vi "ReadALLControlRefs.vi"(8 "error in (no error)":errorcluster, 11 "CtlLookup In":T1) -> (0 "error out":errorcluster, 1 "CtlRef Array":refnum<vi>[](array[refnum]), 2 "CtlName Array":string[](array[string]), 3 "CtlLookup Out":T1)   [LabVIEW 2018, in "CtlReferences.lvlib" / "CtlReferences.lvclass"]
doc: "Read all Refs from DVR"
uses:
  CtlReferences.lvclass
  TypeDefs/CtlLookup.ctl
  CtlReferences.lvclass/CtlReferences.ctl
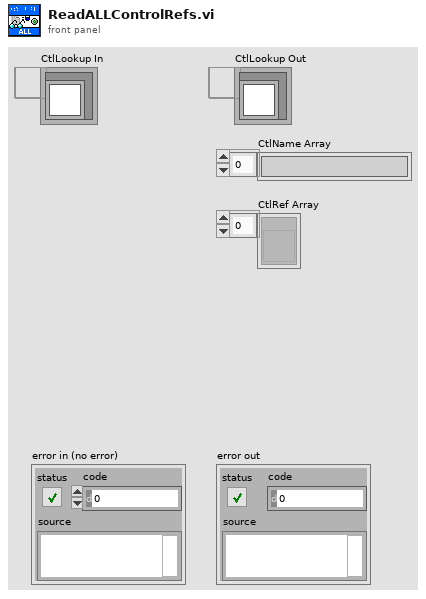
[diagram p1: front panel]
types:
  T1 = typedef "CtlReferences.lvlib/CtlReferences.lvclass/CtlLookup.ctl" = refnum<data-value>
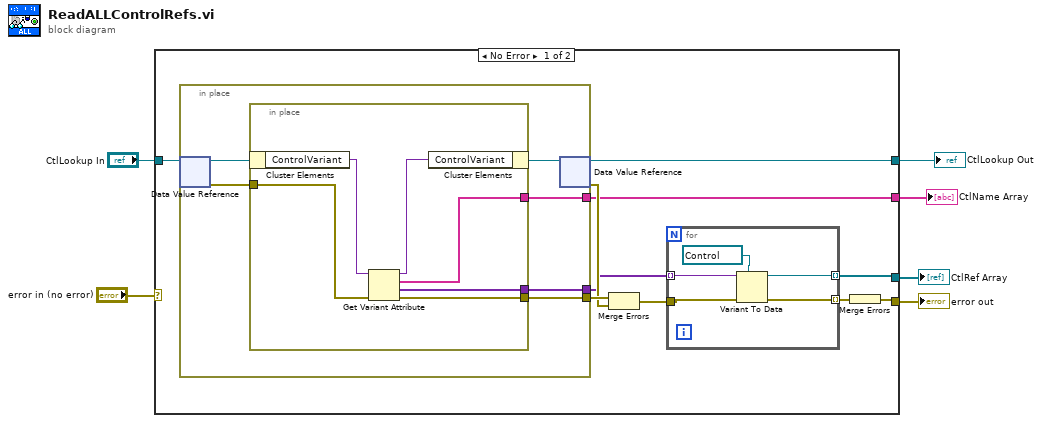
[diagram p0: block diagram]
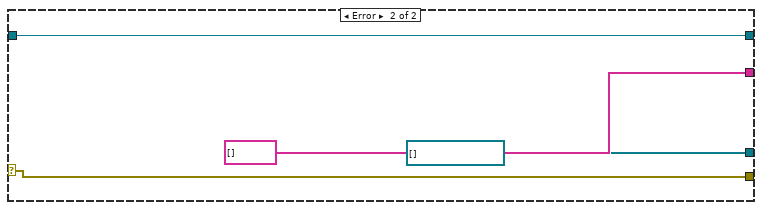
[diagram p2: hidden frame]
diagram:
  n1 = case shown="No Error" "error in (no error)" {
    selector: "error in (no error)" -> [_ w37]
    tunnel: "CtlLookup In" -> [w16 w35]
    tunnel: [w7 w37] -> w1
    tunnel: [w13 string[] []] -> w4
    tunnel: [w12 w35] -> w6
    tunnel: [w8 refnum<vi>[] []] -> w2
    frame No Error {
      n2 = in-place {
        in-place-border: [w26] -> w13
        in-place-border: [w25] -> w9
        in-place-border: [w24] -> w15
        n3 = in-place-dvr #1(w16) -> (w23:refnum<class "CtlReferences.lvclass">, w27:errorcluster)
        n4 = in-place {
          in-place-border: w27 -> [w33]
          in-place-border: [w32] -> w26
          in-place-border: [w31] -> w25
          in-place-border: [w30] -> w24
          n5 = in-place-cluster #2(w23) -> ("ControlVariant"=w29:variant)
          n6 = Get Variant Attribute(Variant=w29, error in=w33) -> (duplicate Variant=w28:variant, names=w32:string[], values=w31:variant[], error out=w30:errorcluster)  [unwired: 2 in]
          n7 = in-place-cluster #2("ControlVariant"=w28) -> (w22:refnum<class "CtlReferences.lvclass">)
        }
        n8 = in-place-dvr #1(w22) -> (w12:T1, w14:errorcluster)
      }
      n9 = Merge Errors(w15, w14) -> (w11:errorcluster)
      n10 = for {
        tunnel: w11 -> [w21]
        tunnel: [w20] -> w10 mode=indexing
        tunnel: w9 -> [w19] mode=indexing
        tunnel: [w17] -> w8 mode=indexing
        n11 = Variant To Data(error in=w21, type=refnum<vi> refnum ("CtlRef"), Variant=w19) -> (data=w17:refnum<vi>, error out=w20:errorcluster)
      }
      n12 = Merge Errors(w10) -> (w7:errorcluster)
    }
    frame Error {
    }
  }
  "CtlLookup Out" <- w6
  "CtlName Array" <- w4
  "error out" <- w1
  "CtlRef Array" <- w2
